vi "Ball and Beam(With Low Pass Fifter)2.vi"() -> ()   [LabVIEW 2011]
uses:
  <vilib>/Utility/file.llb/Write To Spreadsheet File (DBL).vi
  Instance           1 43Saved   Ball and Beam(With Low Pass Fifter) .vi
  Instance           2 43Saved   Ball and Beam(With Low Pass Fifter) .vi
panel:
  in  "file path (dialog if empty)":path
  in  "Ki":dbl=5.0
  out "Theta Output":dbl
  out "X Error":dbl
  out "X Error":dbl(graph)=-0.6885397082002527
  in  "Theta Bound":dbl=3.0
  in  "Kp":dbl=0.5
  in  "Kd":dbl
  in  "X disire":dbl
  out "Vout":dbl
  in  "Vout Bound":dbl=4.5
  in  "Kp1":dbl=5.0
  in  "Sampling rate(Hz)":dbl=50.0
  out "Theta":dbl
  in  "t offset":dbl=-338.2
  in  "t amp":dbl=45.0
  out "Position":dbl
  in  "x offset":dbl=96.61
  in  "x amp":dbl=-21.47
  out "Theta voltage":dbl
  out "X voltage":dbl
  in  "stop":bool
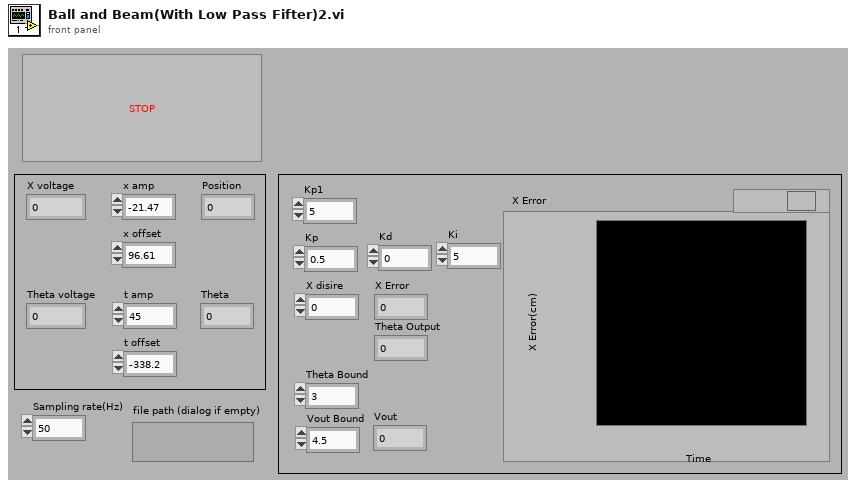
[diagram p1: front panel]
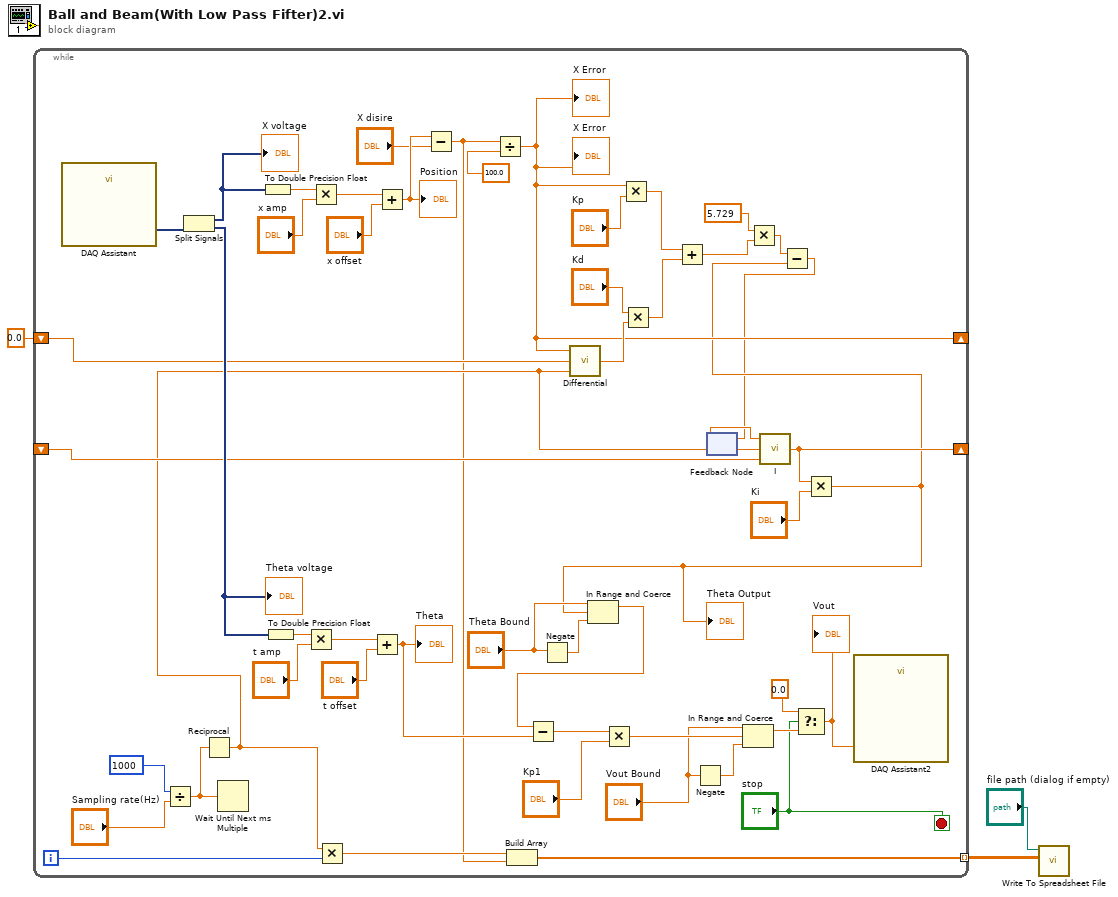
[diagram p0: block diagram]
diagram:
  n1 = while {
    shift-right: [w11] -> _
    shift-left: 0.0 -> [w25]
    shift-right: [w17] -> _
    shift-left: _ -> [w18]
    tunnel: [w9] -> w1 mode=indexing
    i -> [w14]
    stop <- "stop" stop-if-true
    n2 = call "DAQ Assistant"() -> ("data"=w50:dynamicdata)  [unwired: 17 in, 2 out]
    n3 = Divide(x=1000, y="Sampling rate(Hz)") -> (x/y=w31:dbl)
    n4 = Split Signals(w50) -> (w49:dynamicdata, w44:dynamicdata)  [unwired: 2 in]
    "X voltage" <- w49
    "Theta voltage" <- w44
    n5 = Reciprocal(x=w31) -> (1/x=w15:dbl)
    n6 = Wait Until Next ms Multiple(millisecond multiple=w31) -> ()  [unwired: 1 out]
    n7 = To Double Precision Float(number=w49) -> (double precision float=w54:dbl)
    n8 = To Double Precision Float(number=w44) -> (double precision float=w48:dbl)
    n9 = Multiply(x=w48, y="t amp") -> (x*y=w47:dbl)
    n10 = Multiply(x=w54, y="x amp") -> (x*y=w53:dbl)
    n11 = Multiply(x=w15, y=w14) -> (x*y=w13:dbl)
    n12 = Add(x=w47, y="t offset") -> (x+y=w34:dbl)
    "Theta" <- w34
    n13 = Add(x=w53, y="x offset") -> (x+y=w21:dbl)
    "Position" <- w21
    n14 = Subtract(x=w21, y="X disire") -> (x-y=w10:dbl)
    n15 = Divide(x=w10, y=100.0) -> (x/y=w11:dbl)
    "X Error" <- w11
    "X Error" <- w11
    n16 = Build Array(w13, w10) -> (w9:dbl[])
    n17 = Negate(x="Theta Bound") -> (-x=w23:dbl)
    n18 = call "Differential.vi"("Ts"=w15, "X[k-1]"=w25, "X[k]"=w11) -> ("dX"=w30:dbl)
    n19 = Multiply(x=w11, y="Kp") -> (x*y=w27:dbl)
    n20 = Multiply(x="Kd", y=w30) -> (x*y=w26:dbl)
    n21 = Add(x=w27, y=w26) -> (x+y=w5:dbl)
    n22 = Negate(x="Vout Bound") -> (-x=w39:dbl)
    n23 = feedback #1() -> (w16:dbl)  [unwired: 1 in]
    n24 = Multiply(x=5.729 ("y"), y=w5) -> (x*y=w4:dbl)
    n25 = call "I.vi"("sum[k-1]"=w18, "Ts"=w15, "error"=w16) -> ("sum"=w17:dbl)
    n26 = Multiply(x=w17, y="Ki") -> (x*y=w8:dbl)
    "Theta Output" <- w8
    n27 = In Range and Coerce(upper limit="Theta Bound", x=w8, lower limit=w23) -> (coerced(x)=w22:dbl)  [unwired: 1 out]
    n28 = Subtract(x=w22, y=w34) -> (x-y=w32:dbl)
    n29 = Multiply(x=w32, y="Kp1") -> (x*y=w38:dbl)
    n30 = In Range and Coerce(upper limit="Vout Bound", x=w38, lower limit=w39) -> (coerced(x)=w37:dbl)  [unwired: 1 out]
    n31 = Subtract(x=w4, y=w8) -> (x-y=w7:dbl)
    n32 = feedback-in #1(w7) -> ()
    n33 = Select(t=0.0, s="stop", f=w37) -> (s? t:f=w33:dbl)
    "Vout" <- w33
    n34 = call "DAQ Assistant2"("data"=w33) -> ()  [unwired: 17 in, 2 out]
  }
  n35 = call-poly <vilib>:"Write To Spreadsheet File.vi"("2D data"=w1, "file path (dialog if empty)"="file path (dialog if empty)") -> ()  [unwired: 6 in, 1 out]
